vi "OCULOGRAMA_IZQUIERDA_DERECHA.vi"() -> ()   [LabVIEW 2016]
uses:
  <vilib>/LabVIEW Interface for Arduino/Type Defs/Board Type.ctl
  <vilib>/LabVIEW Interface for Arduino/LabVIEW Interface for Arduino.lvlib
panel:
  out "ARRIBA":bool
  out "ABAJO":bool
  in  "ARIBA":dbl
  in  "ABAJO":dbl
  in  "stop":bool
  out "Horizontal":dbl(graph) caption="Waveform Chart"
  # "Condicionales"
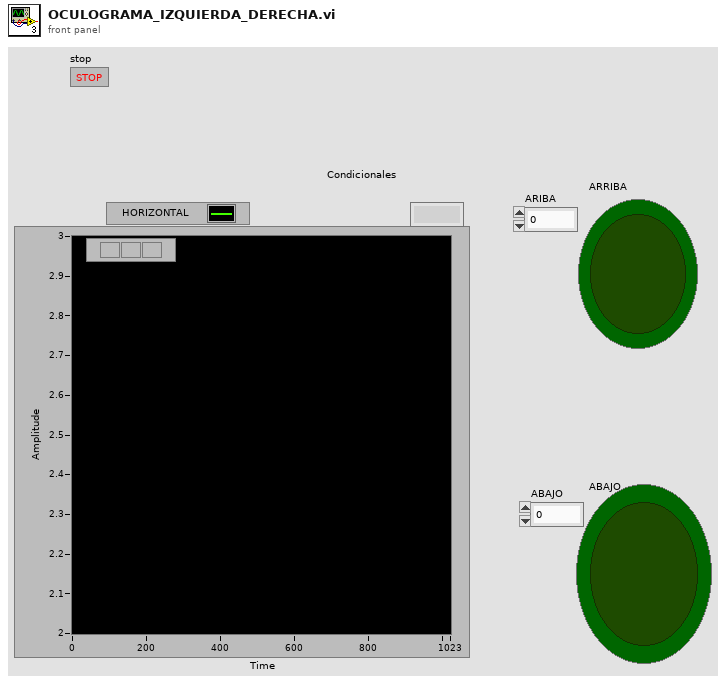
[diagram p1: front panel]
types:
  T1 = typedef "LabVIEW Interface for Arduino.lvlib/Board Type.ctl" = enum16{"Uno", "Dimuelanove w/Atmega 328", "Mega 2560"}
  T2 = typedef "LabVIEW Interface for Arduino.lvlib/Arduino Resource.ctl" = cluster{"VISA resource":refnum<visa-resource-name>, "Board Type":T1, "Connection Type":enum8{"USB / Serial"}, "Bytes Per Packet (15)":u8}
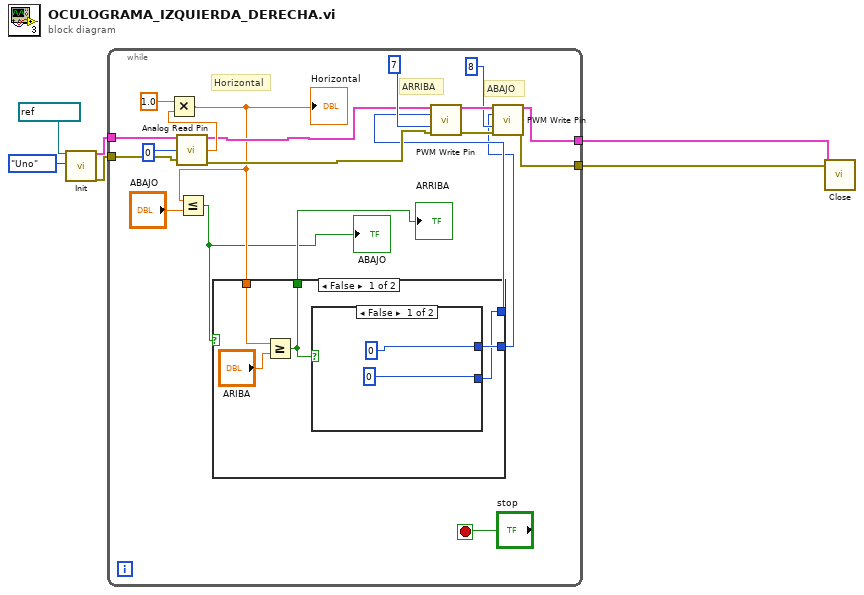
[diagram p0: block diagram]
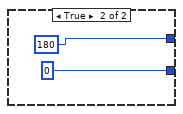
[diagram p2: hidden frame]
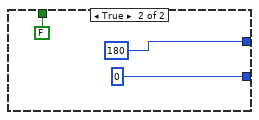
[diagram p3: hidden frame]
diagram:
  n1 = call <vilib>:"Init.vi"("VISA resource"=refnum<visa-resource-name> "COM7", "Board Type (Uno)"=Board_Type."Uno") -> ("Arduino Resource"=w6:T2, "error out"=w5:errorcluster)  [unwired: 16 in]
  n2 = while {
    tunnel: w6 -> [w26]
    tunnel: w5 -> [w25]
    tunnel: [w14] -> w2
    tunnel: [w12] -> w1
    stop <- "stop" stop-if-true
    # "ABAJO"
    # "ARRIBA"
    # "Horizontal"
    n3 = call <vilib>:"Analog Read Pin.vi"("Arduino Resource"=w26, "Analog Input Pin (0)"=u8 0, "error in"=w25) -> ("Arduino Resource"=w15:T2, "Voltage"=w21:dbl, "error out"=w13:errorcluster)  [unwired: 10 in]
    n4 = Multiply(x=1.0, y=w21) -> (x*y=w9:dbl)
    "Horizontal" <- w9
    n5 = Less Or Equal?(x=w9, y="ABAJO") -> (x <= y?=w7:bool)
    "ABAJO" <- w7
    n6 = case shown="False" w7 {
      tunnel: [w27 180] -> w11
      tunnel: [w28 0] -> w10
      tunnel: w9 -> [w31 _]
      tunnel: [w29 FALSE] -> w8
      frame False {
        n7 = Greater Or Equal?(x=w31, y="ARIBA") -> (x >= y?=w29:bool)
        n8 = case shown="False" w29 {
          tunnel: [0 180] -> w28
          tunnel: [0 0] -> w27
          frame False {
          }
          frame True {
          }
        }
      }
      frame True {
      }
    }
    "ARRIBA" <- w8
    n9 = call <vilib>:"PWM Write Pin.vi"("Arduino Resource"=w15, "Duty Cycle (0 - 255)"=w11, "PWM Pin (3)"=u8 7 ("Digital I/O Pin (0)"), "error in"=w13) -> ("Arduino Resource"=w18:T2, "error out"=w16:errorcluster)  [unwired: 10 in]
    n10 = call <vilib>:"PWM Write Pin.vi"("Arduino Resource"=w18, "Duty Cycle (0 - 255)"=w10, "PWM Pin (3)"=u8 8 ("Digital I/O Pin (0)"), "error in"=w16) -> ("Arduino Resource"=w14:T2, "error out"=w12:errorcluster)  [unwired: 10 in]
  }
  n11 = call <vilib>:"Close.vi"("Arduino Resource"=w2, "error in"=w1) -> ()  [unwired: 13 in, 1 out]
